vi "IVA FPGA Image Processing.vi"(0 "Pixel Bus":T2, 1 "Color Plane (Color Plane Extraction 1)":u16(ring) items=["Red", "Green", "Blue"], 7 "Input Valid":bool, 9 "Ready for Output":bool) -> (19 "Ready for Input":bool, 20 "Pixel Bus Out":T1, 27 "Output Valid":bool)   [LabVIEW 2015]
uses:
  <vilib>/visionFPGA/Controls/IMAQ FPGA Pixel Bus RGB32x1.ctl
  <vilib>/visionFPGA/Controls/IMAQ FPGA Pixel Bus u8x1.ctl
  <vilib>/visionFPGA/NI_VDM_FPGA.lvlib
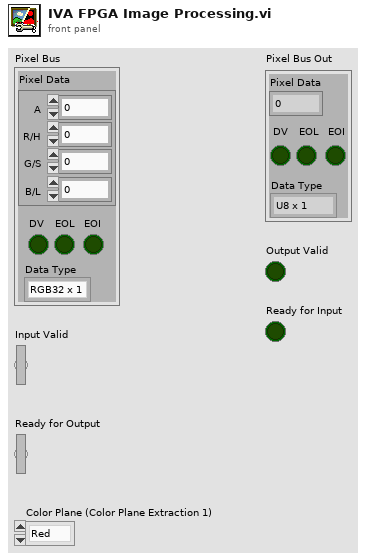
[diagram p1: front panel]
types:
  T1 = typedef "IMAQ FPGA Pixel Bus u8x1.ctl" = cluster{"Pixel Data":u8, "DV":bool, "EOL":bool, "EOI":bool, "Data Type":enum16{"U8 x 1"}}
  T2 = typedef "IMAQ FPGA Pixel Bus RGB32x1.ctl" = cluster{"Pixel Data":cluster{"A":u8, "R/H":u8, "G/S":u8, "B/L":u8}, "DV":bool, "EOL":bool, "EOI":bool, "Data Type":enum16{"RGB32 x 1"}}
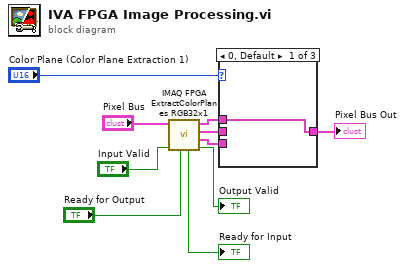
[diagram p0: block diagram]
diagram:
  n1 = call <vilib>:"IMAQ FPGA ExtractColorPlanes RGB32x1.vi"("Ready For Output"="Ready for Output", "Input Valid"="Input Valid", "RGB32 Pixel Bus In"="Pixel Bus") -> ("Output Valid"=→"Output Valid":bool, "Blue Plane Out"=w5:T1, "Green Plane Out"=w6:T1, "Red Plane Out"=w7:T1, "Ready for Input"=→"Ready for Input":bool)  [unwired: 4 in]
  n2 = case shown="0, Default" "Color Plane (Color Plane Extraction 1)" {
    tunnel: [w11 w12 w13] -> w9
    tunnel: w7 -> [w11 _ _]
    tunnel: w6 -> [_ w12 _]
    tunnel: w5 -> [_ _ w13]
    frame 0, Default {
    }
    frame 1 {
    }
    frame 2 {
    }
  }
  "Pixel Bus Out" <- w9
